vi "SD-FindElementStartByName.vi"(6 "offset (0)":i32, 10 "Element Name":string, 11 "string":string) -> (1 "after substring":string, 2 "match substring":string, 3 "before substring":string, 4 "offset past match":i32)   [LabVIEW 2020]
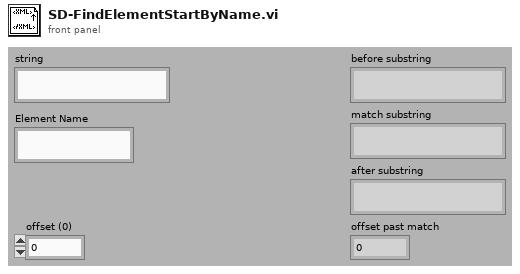
[diagram p1: front panel]
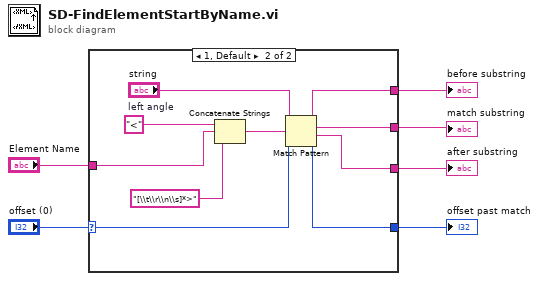
[diagram p0: block diagram]
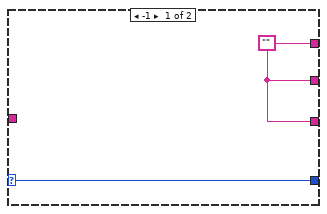
[diagram p2: hidden frame]
diagram:
  n1 = case shown="1, Default" "offset (0)" {
    selector: "offset (0)" -> [w8 w11]
    tunnel: [w7 w15] -> w6
    tunnel: [w7 w14] -> w5
    tunnel: [w8 w13] -> w4
    tunnel: [w7 w12] -> w3
    tunnel: "Element Name" -> [_ w9]
    frame -1 {
      w7 = ""
    }
    frame 1, Default {
      w18 = "<"  # left angle
      n2 = Concatenate Strings(w18, w9, "[\\t\\r\\n\\s]*>" ("regular expression")) -> (w16:string)
      n3 = Match Pattern(string="string", regular expression=w16, offset (0)=w11) -> (before substring=w15:string, match substring=w12:string, after substring=w14:string, offset past match=w13:i32)
    }
  }
  "before substring" <- w6
  "match substring" <- w3
  "after substring" <- w5
  "offset past match" <- w4
